vi "Config Current Range.vi"(0 "VISA resource name":refnum<visa-resource-name>, 5 "A Range (12: 20A)":u16(ring)=12 items=["Auto", "5mA", "10mA", "20mA", "50mA", "100mA", "200mA", "0.5A", "1A", "2A", "5A", "10A", "20A", "50mV", "100mV", "200mV", "2.5V", "5V", "10V"], 11 "error in (no error)":errorcluster) -> (4 "VISA resource name out":refnum<visa-resource-name>, 15 "error out":errorcluster)   [LabVIEW 2013, in "Yokogawa WT200 Series.lvlib"]
doc: "This VI sends the current range command to the WT200 Series."
uses:
  <instrlib>/Yokogawa WT200 Series/Yokogawa WT200 Series.lvlib
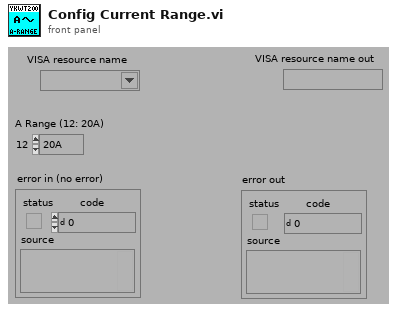
[diagram p1: front panel]
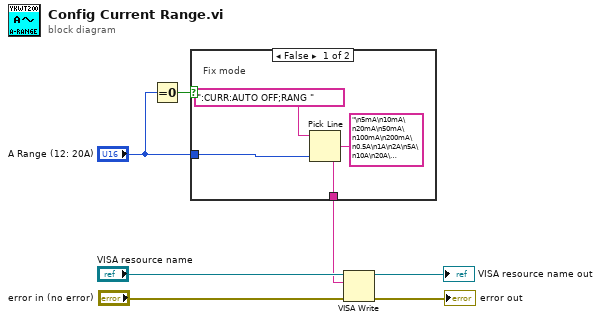
[diagram p0: block diagram]
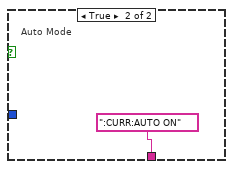
[diagram p2: hidden frame]
diagram:
  n1 = Equal To 0?(x="A Range (12: 20A)") -> (x = 0?=w7:bool)
  n2 = case shown="False" w7 {
    tunnel: [w10 ":CURR:AUTO ON"] -> w1
    tunnel: "A Range (12: 20A)" -> [w8 _]
    frame False {
      # "Fix mode"
      n3 = Pick Line(string ("")=":CURR:AUTO OFF;RANG ", multi-line string="\n5mA\n10mA\n20mA\n50mA\n100mA\n200mA\n0.5A\n1A\n2A\n5A\n10A\n20A\nEXT,50mV\nEXT,100mV\nEXT,200mV\nEXT,2.5V\nEXT,5V\nEXT,10V", line index=w8) -> (output string=w10:string)
    }
    frame True {
      # "Auto Mode"
    }
  }
  n4 = VISA Write(VISA resource name="VISA resource name", write buffer=w1, error in (no error)="error in (no error)") -> (VISA resource name out=→"VISA resource name out":refnum<visa-resource-name>, error out=→"error out":errorcluster)  [unwired: 1 out]
